vi "Get Controls from Tab Recursively.vi"(0 "page sel refnum":refnum<vi>, 11 "error in":errorcluster) -> (4 "indicators in tab":refnum<vi>[](array[refnum]), 6 "controls in tab":refnum<vi>[](array[refnum]), 15 "error out":errorcluster)   [LabVIEW 2021, in "Converter.lvlib"]
uses:
  Converter.lvlib
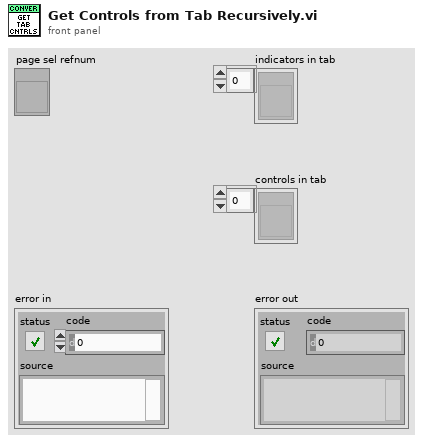
[diagram p1: front panel]
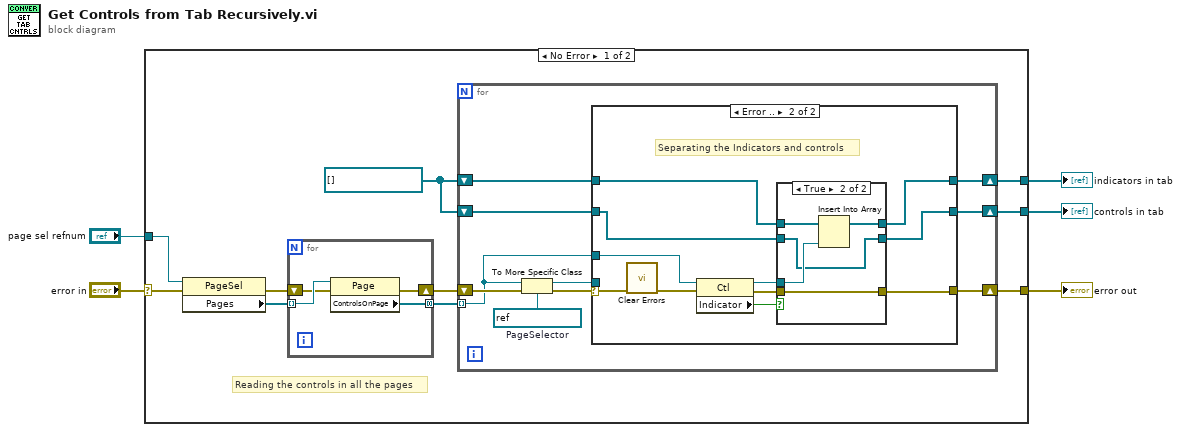
[diagram p0: block diagram]
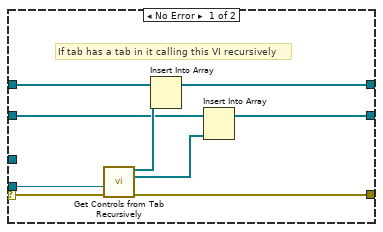
[diagram p2: hidden frame]
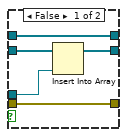
[diagram p3: hidden frame]
diagram:
  n1 = case shown="No Error" "error in" {
    selector: "error in" -> [w13 w60]
    tunnel: "page sel refnum" -> [w15 _]
    tunnel: [w10 _] -> w3
    tunnel: [w9 w60] -> w2
    tunnel: [w7 _] -> w1
    frame No Error {
      w6 = refnum<vi>[] []
      # "Reading the controls in all the pages"
      n2 = property class="PageSel"(reference=w15, error in=w13) -> (error out=w12:errorcluster, "Pages"=w14:refnum<vi>[])  [unwired: 1 out]
      n3 = for {
        tunnel: w14 -> [w59] mode=indexing
        tunnel: [w57] -> w8 mode=concatenating
        shift-right: [w56] -> w11
        shift-left: w12 -> [w58]
        n4 = property class="Page"(reference=w59, error in=w58) -> (error out=w56:errorcluster, "ControlsOnPage"=w57:refnum<vi>[])  [unwired: 1 out]
      }
      n5 = for {
        tunnel: w8 -> [w19] mode=indexing
        shift-right: [w20] -> w10
        shift-left: w6 -> [w22]
        shift-right: [w18] -> w9
        shift-left: w11 -> [w25]
        shift-right: [w16] -> w7
        shift-left: w6 -> [w17]
        w24 = refnum<vi> refnum  # PageSelector
        n6 = To More Specific Class(target class=w24, reference=w19, error in=w25) -> (specific class reference=w21:refnum<vi>, error out=w23:errorcluster)
        n7 = case shown="Error .." w23 {
          selector: w23 -> [w34 w45]
          tunnel: w22 -> [w31 w42]
          tunnel: w21 -> [w33 _]
          tunnel: [w30 w38] -> w20
          tunnel: w19 -> [_ w41]
          tunnel: [w32 w36] -> w18
          tunnel: w17 -> [w28 w39]
          tunnel: [w26 w37] -> w16
          frame No Error {
            # "If tab has a tab in it calling this VI recursively"
            n8 = call "Get Controls from Tab Recursively.vi"("page sel refnum"=w33, "error in"=w34) -> ("indicators in tab"=w29:refnum<vi>[], "controls in tab"=w27:refnum<vi>[], "error out"=w32:errorcluster)  [unwired: 11 in]
            n9 = Insert Into Array(array=w31, new element=w29) -> (w30:refnum<vi>[])  [unwired: 1 in]
            n10 = Insert Into Array(array=w28, new element=w27) -> (w26:refnum<vi>[])  [unwired: 1 in]
          }
          frame Error {
            # "Separating the Indicators and controls"
            n11 = call <vilib>:"Clear Errors.vi"("error in (no error)"=w45) -> ("error out"=w44:errorcluster)  [unwired: 5 in, 1 out]
            n12 = property class="Ctl"(reference=w41, error in=w44) -> (reference out=w40:refnum<vi>, error out=w35:errorcluster, "Indicator"=w43:bool)
            n13 = case shown="True" w43 {
              tunnel: w42 -> [w50 w55]
              tunnel: [w50 w54] -> w38
              tunnel: w40 -> [w48 w53]
              tunnel: w39 -> [w49 w52]
              tunnel: [w47 w52] -> w37
              tunnel: [w46 w51] -> w36
              tunnel: w35 -> [w46 w51]
              frame False {
                n14 = Insert Into Array(array=w49, new element=w48) -> (w47:refnum<vi>[])  [unwired: 1 in]
              }
              frame True {
                n15 = Insert Into Array(array=w55, new element=w53) -> (w54:refnum<vi>[])  [unwired: 1 in]
              }
            }
          }
        }
      }
    }
    frame Error {
    }
  }
  "error out" <- w2
  "indicators in tab" <- w3
  "controls in tab" <- w1
